vi "非均匀DAC.vi"(8 "Vref V":dbl=2.56, 11 "数字编码":dbl[](array[numeric])) -> (3 "x+y 2":dbl)   [LabVIEW 2020]
uses:
  <vilib>/express/express arith-compare/Formula/XNode/ExpressFormulaBlockNode.xnode
panel:
  out "s":dbl
  out "c":dbl
  out "p":dbl
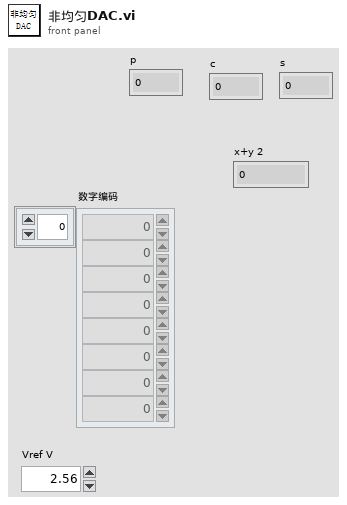
[diagram p1: front panel]
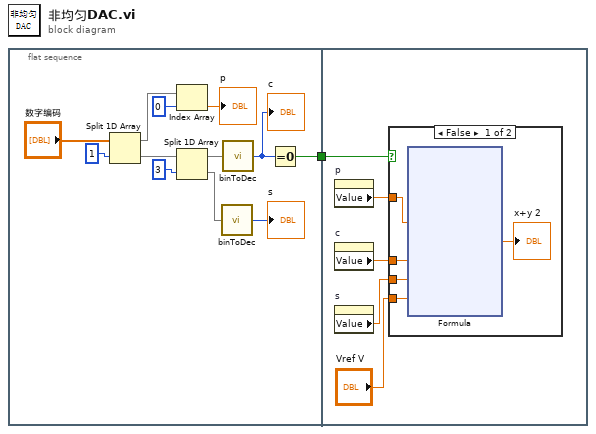
[diagram p0: block diagram]
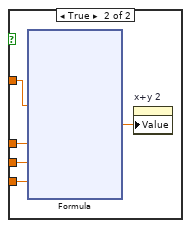
[diagram p2: hidden frame]
diagram:
  n1 = flat-sequence {
    tunnel: [w2] -> w1
    tunnel: w1 -> [w14]
    frame #0 {
      n2 = Split 1D Array(array="数字编码", index=1) -> (first subarray=w11:dbl[], second subarray=w8:dbl[])
      n3 = Index Array(array=w11, index=0) -> (element=→"p":dbl)
      n4 = Split 1D Array(array=w8, index=3) -> (first subarray=w6:dbl[], second subarray=w5:dbl[])
      n5 = call "binToDec.vi"("Array 2"=w5) -> ("output"=→"s":i32)
      n6 = call "binToDec.vi"("Array 2"=w6) -> ("output"=w3:i32)
      "c" <- w3
      n7 = Equal To 0?(x=w3) -> (x = 0?=w2:bool)
    }
    frame #1 {
      n8 = property on="p" class="DigNum (strict)"() -> ("Value"=w15:dbl)  [unwired: 2 in, 2 out]
      n9 = property on="c" class="DigNum (strict)"() -> ("Value"=w16:dbl)  [unwired: 2 in, 2 out]
      n10 = property on="s" class="DigNum (strict)"() -> ("Value"=w17:dbl)  [unwired: 2 in, 2 out]
      n11 = case shown="False" w14 {
        tunnel: w15 -> [w23 w42]
        tunnel: w16 -> [w22 w41]
        tunnel: w17 -> [w21 w40]
        tunnel: "Vref V" -> [w20 w39]
        frame False {
          n12 = xnode "Formula"("p"=w23, "c"=w22, "s"=w21, "Vref"=w20) -> ("Result"=→"x+y 2":dbl)  [unwired: 1 in, 1 out]
        }
        frame True {
          n13 = xnode "Formula"("p"=w42, "c"=w41, "s"=w40, "Vref"=w39) -> ("Result"=w38:dbl)  [unwired: 1 in, 1 out]
          n14 = property on="x+y 2" class="DigNum (strict)"("Value"=w38) -> ()  [unwired: 2 in, 2 out]
        }
      }
    }
  }
